vi "GetChannel.vi"(8 "error in":errorcluster, 10 "index":i32, 11 "T560Session in":refnum<class "T560Session.lvclass">) -> (0 "error out":errorcluster, 2 "T560Channel.lvclass":refnum<class "T560Channel.lvclass">, 3 "T560Session out":refnum<class "T560Session.lvclass">)   [LabVIEW 2013, in "T560Session.lvclass"]
uses:
  T560Session.lvclass
  T560ChannelClass/T560Channel.lvclass
  T560Session.lvclass/T560Session.ctl
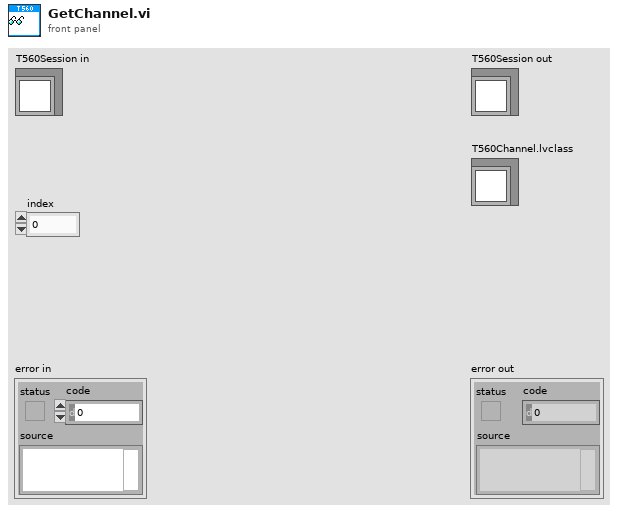
[diagram p1: front panel]
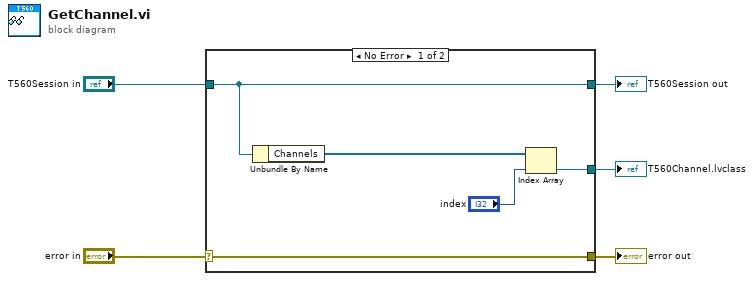
[diagram p0: block diagram]
diagram:
  n1 = case shown="No Error" "error in" {
    selector: "error in" -> [w10 w11]
    tunnel: [w10 w11] -> w4
    tunnel: [w9 w12] -> w2
    tunnel: "T560Session in" -> [w9 w12]
    tunnel: [w6 _] -> w1
    frame No Error {
      n2 = Unbundle By Name(w9) -> ("Channels"=w8:refnum<class "T560Channel.lvclass">[])
      n3 = Index Array(array=w8, index="index") -> (element=w6:refnum<class "T560Channel.lvclass">)
    }
    frame Error {
    }
  }
  "error out" <- w4
  "T560Session out" <- w2
  "T560Channel.lvclass" <- w1
